vi "calculate Volath4 function.vi"(8 "error in (no error)":errorcluster, 11 "Autofocus in":refnum<class "Autofocus.lvclass">) -> (0 "error out":errorcluster, 3 "Autofocus out":refnum<class "Autofocus.lvclass">)   [LabVIEW 2012, in "Autofocus.lvclass"]
uses:
  Autofocus.lvclass
  Sharpness Measure.ctl
  Autofocus.lvclass/Autofocus.ctl
  <vilib>/Analysis/baseanly.llb/Mean (DBL).vi
  <vilib>/Utility/file.llb/Write To Spreadsheet File (DBL).vi
  <vilib>/Utility/file.llb/Write To Spreadsheet File (string).vi
  <vilib>/Analysis/NI_AALBase.lvlib
panel:
  out "total time":u32
  out "mean calculation time per image":dbl format="%0.2f"
  in  "Image to select ROI":path
  in  "ROI?":bool
  out "Image Source":T1(plugin-control)
  out "Number of Files found in fodler":i32
  out "Array":dbl[](array[numeric])
  in  "File Path":path
  in  "Sharpness measure":T2
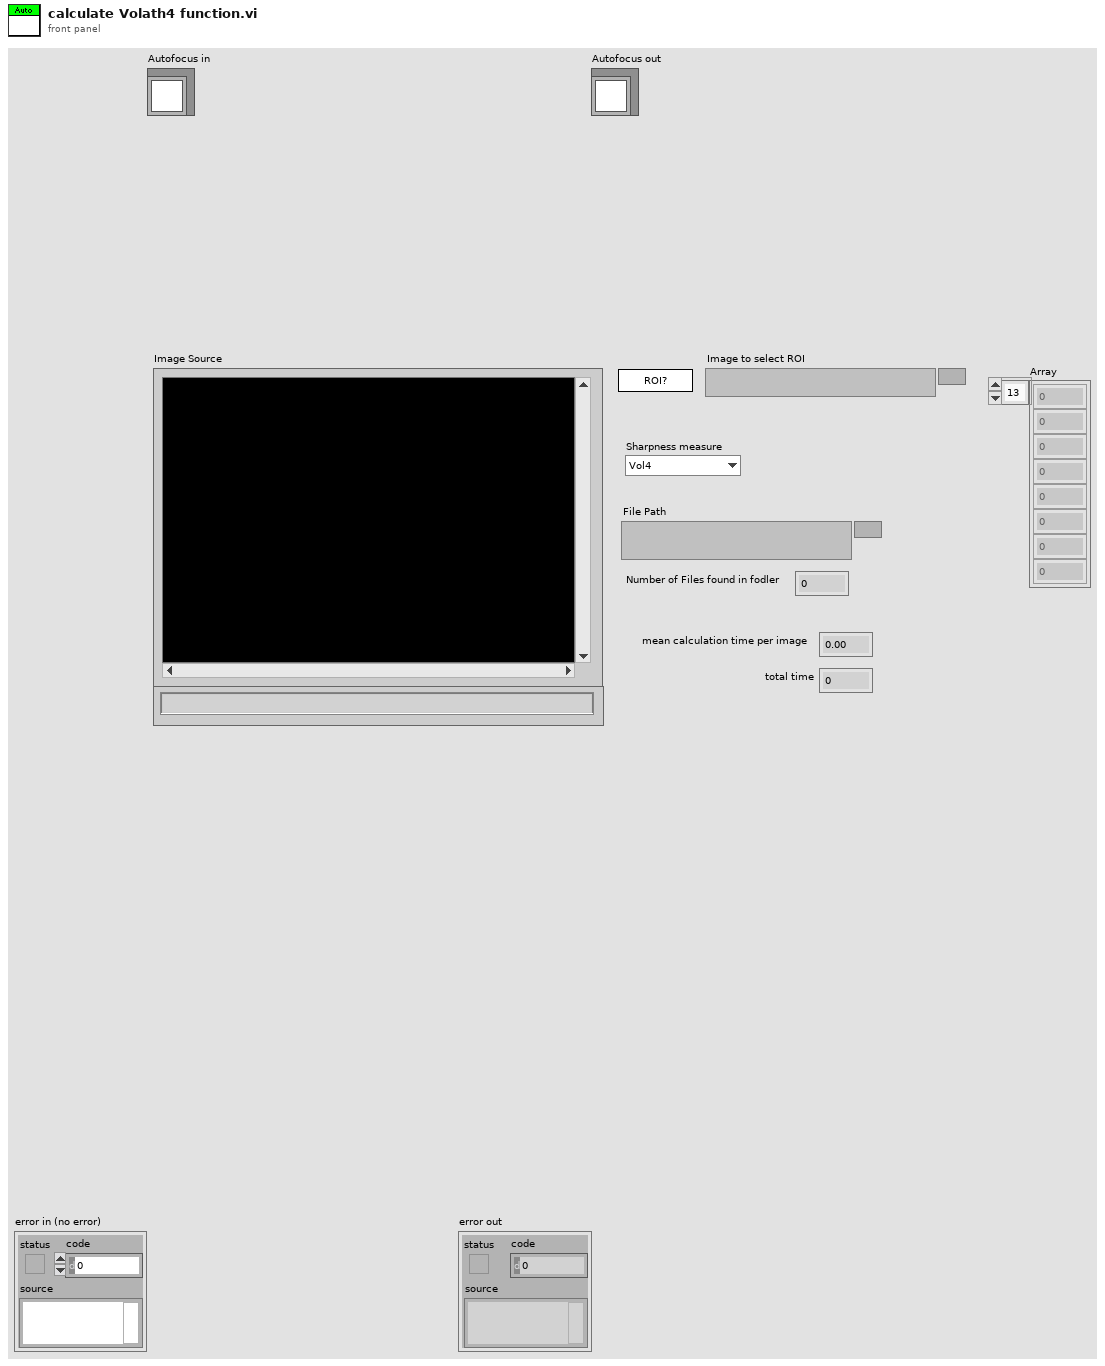
[diagram p1: front panel]
types:
  T1 = typedef "IMAQ Image.ctl" = refnum<image>
  T2 = typedef "Autofocus.lvclass/Sharpness Measure.ctl" = enum16{"Vol4", "Gradient Square"}
  T3 = typedef "Image Type" = u32
  T4 = typedef "ROI Descriptor" = cluster{"Global Rectangle":i32[], "Contours":cluster{"ID":enum32{"External", "Internal"}, "Type":u32, "Coordinates":i32[]}[]}
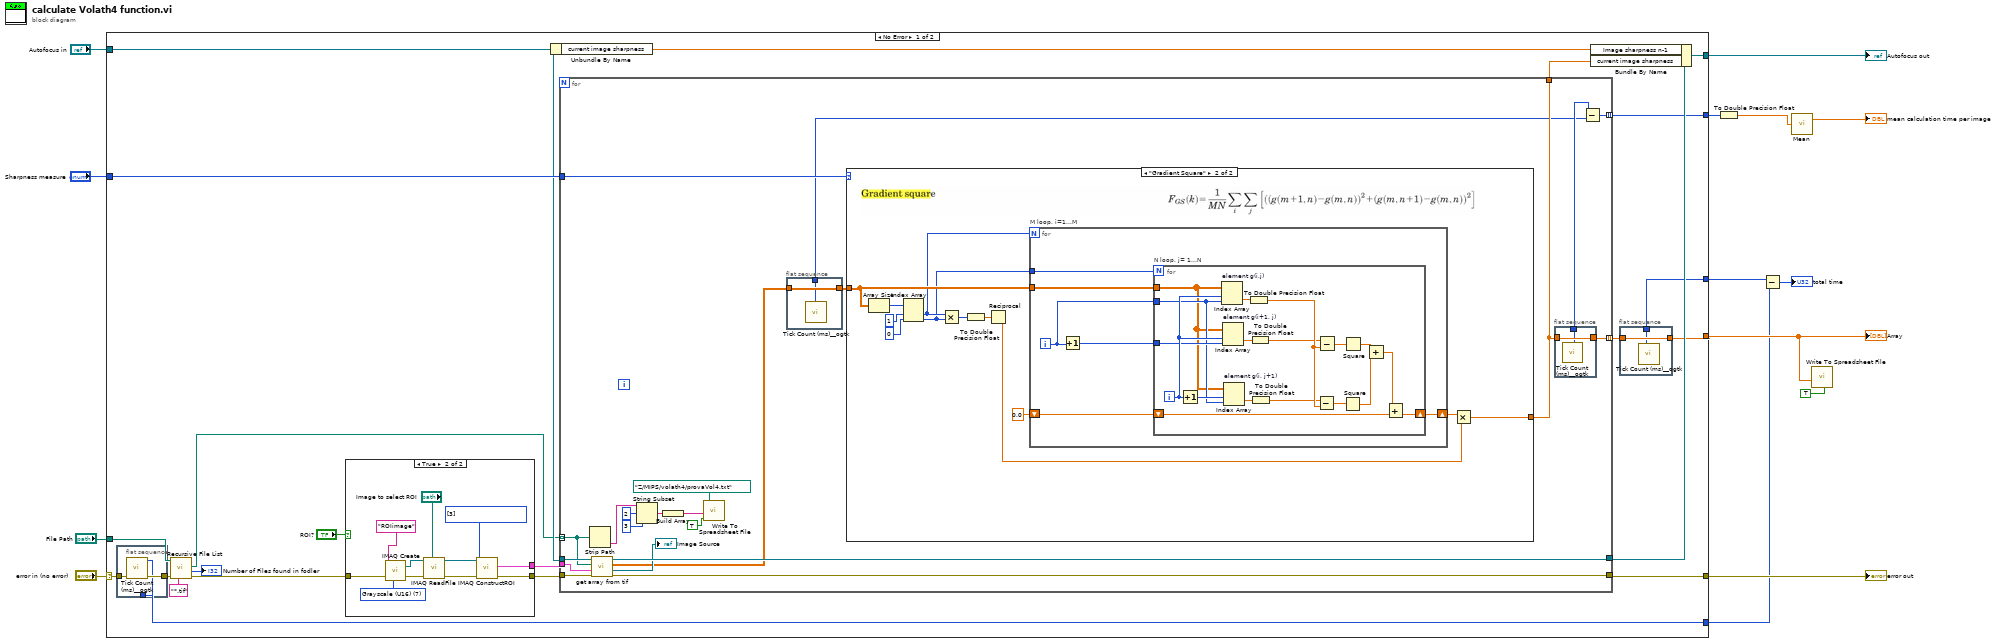
[diagram p0: block diagram]
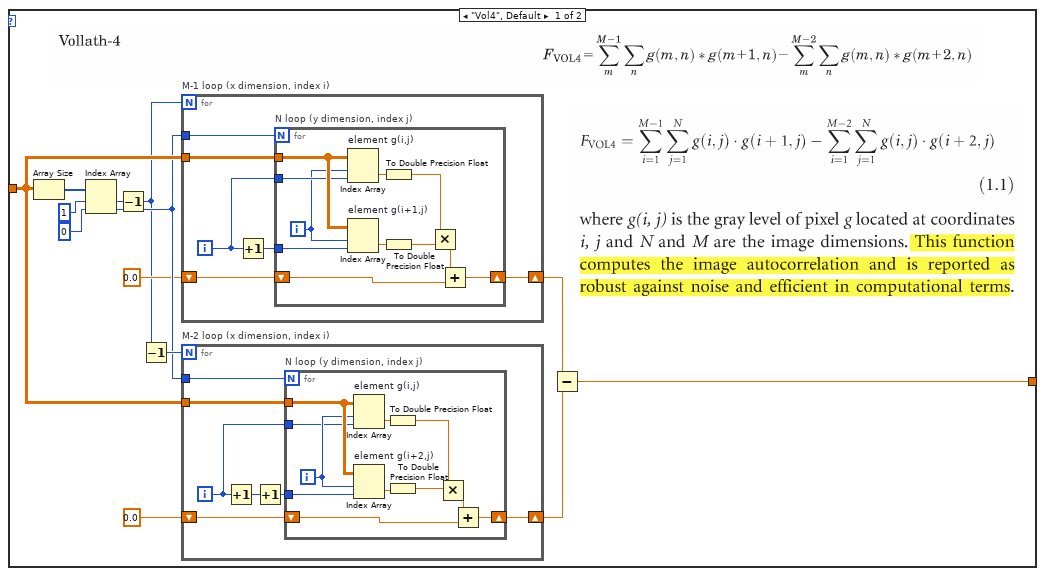
[diagram p3: hidden frame]
diagram:
  n1 = case shown="No Error" "error in (no error)" {
    selector: "error in (no error)" -> [w21 w165]
    tunnel: [w34 w165] -> w13
    tunnel: [w31 w164] -> w11
    tunnel: "Autofocus in" -> [w33 w164]
    tunnel: "Sharpness measure" -> [w35 _]
    tunnel: "File Path" -> [w30 _]
    tunnel: [w19 _] -> w8
    tunnel: [w17 _] -> w2
    tunnel: [w16 _] -> w6
    tunnel: [w15 _] -> w3
    frame No Error {
      n2 = flat-sequence {
        tunnel: w21 -> [w41]
        tunnel: [w40] -> w20
        tunnel: [w39] -> w15
        frame #0 {
          n3 = call <userlib>:"Tick Count (ms)__ogtk.vi"("error in (no error)"=w41) -> ("error out"=w40:errorcluster, "millisecond timer value"=w39:u32)  [unwired: 9 in]
        }
      }
      n4 = call <vilib>:"Recursive File List.vi"("pattern"="*.tif", "error in (no error)"=w20, "Folder Path"=w30) -> ("error out"=w26:errorcluster, "Number of Files"=→"Number of Files found in fodler":i32, "All Files in Dir"=w23:path[])  [unwired: 4 in, 2 out]
      n5 = case shown="True" "ROI?" {
        tunnel: w26 -> [w42 w53]
        tunnel: [w42 w52] -> w25
        tunnel: [_ w51] -> w24
        frame False {
        }
        frame True {
          w48 = T3 7 items=["Grayscale (U8)", "Grayscale (I16)", "Grayscale (SGL)", "Complex (CSG)", "RGB (U32)", "HSL (U32)", "RGB (U64)", "Grayscale (U16)"] ("Image Type")
          w50 = u32[] [3] items=["No Selection", "Point", "Line", "Rectangle", "Oval", "Polygon", "Freehand Region", "Annulus", "Zoom", "Pan", "Broken Line", "Freehand Line", "Rotated Rectangle"] ("Tools")
          n6 = call "IMAQ Create"("Image Name"="ROIimage", "Image Type"=w48, "error in (no error)"=w53) -> ("New Image"=w49:T1, "error out"=w46:errorcluster)  [unwired: 2 in]
          n7 = call "IMAQ ReadFile"("File Path"="Image to select ROI", "error in (no error)"=w46, "Image"=w49) -> ("error out"=w45:errorcluster, "Image Out"=w44:T1)  [unwired: 4 in, 3 out]
          n8 = call "IMAQ ConstructROI"("error in (no error)"=w45, "Tools"=w50, "Image"=w44) -> ("error out"=w52:errorcluster, "ROI Descriptor Out"=w51:T4)  [unwired: 5 in, 2 out]
        }
      }
      n9 = Unbundle By Name(w33) -> ("current image sharpness"=w36:dbl)
      n10 = for {
        tunnel: [w57] -> w28
        tunnel: w35 -> [w75]
        tunnel: w25 -> [w74]
        tunnel: [w73] -> w34
        tunnel: w33 -> [w72]
        tunnel: [w71] -> w32
        tunnel: w23 -> [w68] mode=indexing
        tunnel: [w58] -> w18 mode=indexing
        tunnel: w24 -> [w61]
        tunnel: [w54] -> w16 mode=indexing
        n11 = Strip Path(path=w68) -> (name=w66:string)  [unwired: 1 out]
        n12 = call-dynamic "get array from tif.vi"("error in (no error)"=w74, "ROI Descriptor Out"=w61, "File Path"=w68, "Autofocus in"=w72) -> ("error out"=w73:errorcluster, "Image Source"=→"Image Source":T1, "Array"=w59:dbl[][], "Autofocus out"=w71:refnum<class "Autofocus.lvclass">)  [unwired: 4 in]
        n13 = String Subset(string=w66, offset (0)=2, length (rest)=3 ("length (rest)")) -> (substring=w65:string)
        n14 = Build Array(w65) -> (w67:string[])
        n15 = call-poly <vilib>:"Write To Spreadsheet File.vi"("append to file? (new file:F)"=TRUE, "1D data"=w67, "file path (dialog if empty)"=path "Z:/MIPS/volath4/provaVol4.txt") -> ()  [unwired: 5 in, 1 out]
        n16 = flat-sequence {
          tunnel: [w79] -> w60
          tunnel: w59 -> [w79]
          tunnel: [w78] -> w55
          frame #0 {
            n17 = call <userlib>:"Tick Count (ms)__ogtk.vi"() -> ("millisecond timer value"=w78:u32)  [unwired: 10 in, 1 out]
          }
        }
        n18 = case shown="\"Gradient Square\"" w75 {
          tunnel: w60 -> [w87 w136]
          tunnel: [w81 w131] -> w57
          frame "Vol4", Default {
            n19 = Array Size(array=w87) -> (size(s)=w92:i32[])
            n20 = Index Array(array=w92, index #1=1 ("index"), index #2=0 ("index")) -> (element #1=w88:i32, element #2=w86:i32)
            n21 = Decrement(x=w88) -> (x-1=w80:i32)
            n22 = Decrement(x=w80) -> (x-1=w89:i32)
            n23 = for "M-1 loop (x dimension, index i)" {
              N: w80 -> [_]
              tunnel: w87 -> [w116]
              tunnel: w86 -> [w115]
              shift-right: [w112] -> w85
              shift-left: 0.0 -> [w111]
              i -> [w114]
              n24 = Increment(x=w114) -> (x+1=w113:i32)
              n25 = for "N loop (y dimension, index j)" {
                N: w115 -> [_]
                tunnel: w116 -> [w126]
                shift-right: [w119] -> w112
                shift-left: w111 -> [w127]
                tunnel: w114 -> [w124]
                tunnel: w113 -> [w122]
                i -> [w123]
                n26 = Index Array "element g(i,j)"(array=w126, index (row)=w123, index (col)=w124) -> (element=w121:dbl)
                n27 = Index Array "element g(i+1,j)"(array=w126, index (row)=w123, index (col)=w122) -> (element=w120:dbl)
                n28 = To Double Precision Float(number=w121) -> (double precision float=w117:dbl)
                n29 = To Double Precision Float(number=w120) -> (double precision float=w118:dbl)
                n30 = Multiply(x=w117, y=w118) -> (x*y=w125:dbl)
                n31 = Add(x=w125, y=w127) -> (x+y=w119:dbl)
              }
            }
            n32 = for "M-2 loop (x dimension, index i)" {
              N: w89 -> [_]
              tunnel: w87 -> [w98]
              tunnel: w86 -> [w99]
              shift-right: [w94] -> w84
              shift-left: 0.0 -> [w93]
              i -> [w97]
              n33 = Increment(x=w97) -> (x+1=w96:i32)
              n34 = Increment(x=w96) -> (x+1=w95:i32)
              n35 = for "N loop (y dimension, index j)" {
                N: w99 -> [_]
                tunnel: w98 -> [w107]
                tunnel: w97 -> [w105]
                tunnel: w95 -> [w104]
                shift-right: [w103] -> w94
                shift-left: w93 -> [w102]
                i -> [w106]
                n36 = Index Array "element g(i,j)"(array=w107, index (row)=w106, index (col)=w105) -> (element=w109:dbl)
                n37 = Index Array "element g(i+2,j)"(array=w107, index (row)=w106, index (col)=w104) -> (element=w110:dbl)
                n38 = To Double Precision Float(number=w109) -> (double precision float=w100:dbl)
                n39 = To Double Precision Float(number=w110) -> (double precision float=w101:dbl)
                n40 = Multiply(x=w100, y=w101) -> (x*y=w108:dbl)
                n41 = Add(x=w108, y=w102) -> (x+y=w103:dbl)
              }
            }
            n42 = Subtract(x=w85, y=w84) -> (x-y=w81:dbl)
          }
          frame "Gradient Square" {
            n43 = Array Size(array=w136) -> (size(s)=w139:i32[])
            n44 = Index Array(array=w139, index #1=1 ("index"), index #2=0 ("index")) -> (element #1=w129:i32, element #2=w128:i32)
            n45 = Multiply(x=w129, y=w128) -> (x*y=w135:i32)
            n46 = To Double Precision Float(number=w135) -> (double precision float=w134:dbl)
            n47 = Reciprocal(x=w134) -> (1/x=w130:dbl)
            n48 = for "M loop, i=1...M" {
              N: w129 -> [_]
              tunnel: w136 -> [w145]
              tunnel: w128 -> [w144]
              shift-right: [w141] -> w132
              shift-left: 0.0 -> [w140]
              i -> [w143]
              n49 = Increment(x=w143) -> (x+1=w142:i32)
              n50 = for "N loop, j= 1...N" {
                N: w144 -> [_]
                tunnel: w145 -> [w159]
                tunnel: w143 -> [w160]
                tunnel: w142 -> [w162]
                shift-right: [w149] -> w141
                shift-left: w140 -> [w151]
                i -> [w163]
                n51 = Increment(x=w163) -> (x+1=w161:i32)
                n52 = Index Array "element g(i,j)"(array=w159, index (row)=w163, index (col)=w160) -> (element=w154:dbl)
                n53 = Index Array "element g(i+1, j)"(array=w159, index (row)=w163, index (col)=w162) -> (element=w158:dbl)
                n54 = Index Array "element g(i, j+1)"(array=w159, index (row)=w161, index (col)=w160) -> (element=w155:dbl)
                n55 = To Double Precision Float(number=w154) -> (double precision float=w148:dbl)
                n56 = To Double Precision Float(number=w158) -> (double precision float=w147:dbl)
                n57 = To Double Precision Float(number=w155) -> (double precision float=w146:dbl)
                n58 = Subtract(x=w146, y=w148) -> (x-y=w156:dbl)
                n59 = Subtract(x=w147, y=w148) -> (x-y=w157:dbl)
                n60 = Square(x=w156) -> (x^2=w152:dbl)
                n61 = Square(x=w157) -> (x^2=w153:dbl)
                n62 = Add(x=w153, y=w152) -> (x+y=w150:dbl)
                n63 = Add(x=w150, y=w151) -> (x+y=w149:dbl)
              }
            }
            n64 = Multiply(x=w132, y=w130) -> (x*y=w131:dbl)
          }
        }
        n65 = flat-sequence {
          tunnel: [w77] -> w58
          tunnel: w57 -> [w77]
          tunnel: [w76] -> w56
          frame #0 {
            n66 = call <userlib>:"Tick Count (ms)__ogtk.vi"() -> ("millisecond timer value"=w76:u32)  [unwired: 10 in, 1 out]
          }
        }
        n67 = Subtract(x=w56, y=w55) -> (x-y=w54:u32)
      }
      n68 = Bundle By Name(cluster=w32, "Image sharpness n-1"=w36, "current image sharpness"=w28) -> (w31:refnum<class "Autofocus.lvclass">)
      n69 = flat-sequence {
        tunnel: [w38] -> w19
        tunnel: w18 -> [w38]
        tunnel: [w37] -> w17
        frame #0 {
          n70 = call <userlib>:"Tick Count (ms)__ogtk.vi"() -> ("millisecond timer value"=w37:u32)  [unwired: 10 in, 1 out]
        }
      }
    }
    frame Error {
    }
  }
  "error out" <- w13
  "Autofocus out" <- w11
  "Array" <- w8
  n71 = To Double Precision Float(number=w6) -> (double precision float=w5:dbl[])
  n72 = Subtract(x=w2, y=w3) -> (x-y=→"total time":u32)
  n73 = call-poly <vilib>:"Mean.vi"("X"=w5) -> ("mean"=→"mean calculation time per image":dbl)  [unwired: 1 out]
  n74 = call-poly <vilib>:"Write To Spreadsheet File.vi"("transpose? (no:F)"=TRUE, "1D data"=w8) -> ()  [unwired: 6 in, 1 out]
